vi "observacao.vi"() -> ()   [LabVIEW 2012] (continued)
                    n1498 = property on="Strong" class="Bool (strict)"("Disabled"=w1912) -> ()  [unwired: 2 in, 2 out]
                    n1499 = property on="WeakSel" class="Bool (strict)"("Value"=w1911) -> ()  [unwired: 2 in, 2 out]
                    n1500 = property on="MediumSel" class="Bool (strict)"("Value"=w1913) -> ()  [unwired: 2 in, 2 out]
                    n1501 = property on="StrongSel" class="Bool (strict)"("Value"=w1911) -> ()  [unwired: 2 in, 2 out]
                    n1502 = property on="Coude" class="Bool (strict)"("DisabledEnum"=w1912) -> ()  [unwired: 2 in, 2 out]
                    n1503 = property on="CoudeSel" class="Bool (strict)"("Value"=w1911) -> ()  [unwired: 2 in, 2 out]
                    n1504 = call "Monta Comando.vi"("Comando"=w1914, "Dispositivo"="FLAT_LO", "Controlador"=w1910) -> ()  [unwired: 4 in, 3 out]
                  }
                  frame True {
                    w1925 = FALSE ("Medium")
                    n1505 = Get Date/Time In Seconds() -> (seconds since 1Jan1904=w1928:timestamp)
                    n1506 = Add(x=w1928, y=10.0) -> (x+y=w1929:timestamp)
                    n1507 = local write "alarm Time"(w1929) -> ()
                    n1508 = property on="Mensage Alarme" class="Str"("Visible"=TRUE) -> ()  [unwired: 2 in, 2 out]
                    n1509 = local write "Flag Alarm"(TRUE ("Flag Alarm")) -> ()
                    n1510 = property on="Medium" class="Bool (strict)"("Value"=w1925) -> ()  [unwired: 2 in, 2 out]
                    n1511 = property on="MediumSel" class="Bool (strict)"("Value"=w1925) -> ()  [unwired: 2 in, 2 out]
                  }
                }
              }
              event "Strong": Value Change {
                w1932 = u16 6 items=["Alarme", "Atencao", "Erro", "Ocupado", "TBD", "LCB", "Trapeira", "Paravento", "DomoRap", "DomoCW", "DomoCCW", "TBD", "Em movimento", "TBD"] ("NomeStatus")
                n1512 = event-data() -> ("NewVal"=w1933:bool)  [unwired: 1 in, 5 out]
                n1513 = call "Bit Status CUP.vi"("NomeStatus"=w1932) -> ("StatBit"=w1931:bool)
                n1514 = case shown="False" w1931 {
                  tunnel: w1933 -> [w1941 _]
                  frame False {
                    w1934 = u16 4 items=["ZERO", "AH", "DEC", "TUBO", "CUP"] ("Controlador")
                    n1515 = case shown="True" w1941 {
                      tunnel: [FALSE w1949] -> w1936
                      tunnel: [w1942 w1949] -> w1940
                      tunnel: [0 2] -> w1937
                      tunnel: ["DESLIGAR" "LIGAR"] -> w1939
                      tunnel: [w1942 TRUE] -> w1938
                      frame False {
                        w1942 = FALSE
                      }
                      frame True {
                        w1949 = FALSE
                        n1516 = local write "DOME"(FALSE) -> ()
                        n1517 = local write "StatShutter"("Busy to Close" ("Status")) -> ()
                      }
                    }
                    n1518 = property on="Medium" class="Bool (strict)"("Disabled"=w1937) -> ()  [unwired: 2 in, 2 out]
                    n1519 = property on="Weak" class="Bool (strict)"("Disabled"=w1937) -> ()  [unwired: 2 in, 2 out]
                    n1520 = property on="Coude" class="Bool (strict)"("DisabledEnum"=w1937) -> ()  [unwired: 2 in, 2 out]
                    n1521 = property on="WeakSel" class="Bool (strict)"("Value"=w1940) -> ()  [unwired: 2 in, 2 out]
                    n1522 = property on="MediumSel" class="Bool (strict)"("Value"=w1936) -> ()  [unwired: 2 in, 2 out]
                    n1523 = property on="StrongSel" class="Bool (strict)"("Value"=w1938) -> ()  [unwired: 2 in, 2 out]
                    n1524 = property on="CoudeSel" class="Bool (strict)"("Value"=w1936) -> ()  [unwired: 2 in, 2 out]
                    n1525 = call "Monta Comando.vi"("Comando"=w1939, "Dispositivo"="FLAT_HI", "Controlador"=w1934) -> ()  [unwired: 4 in, 3 out]
                  }
                  frame True {
                    w1952 = FALSE ("Strong")
                    n1526 = Get Date/Time In Seconds() -> (seconds since 1Jan1904=w1955:timestamp)
                    n1527 = Add(x=w1955, y=10.0) -> (x+y=w1956:timestamp)
                    n1528 = local write "alarm Time"(w1956) -> ()
                    n1529 = property on="Mensage Alarme" class="Str"("Visible"=TRUE) -> ()  [unwired: 2 in, 2 out]
                    n1530 = local write "Flag Alarm"(TRUE ("Flag Alarm")) -> ()
                    n1531 = property on="StrongSel" class="Bool (strict)"("Value"=w1952) -> ()  [unwired: 2 in, 2 out]
                    n1532 = property on="Strong" class="Bool (strict)"("Value"=w1952) -> ()  [unwired: 2 in, 2 out]
                  }
                }
              }
              event "Coude": Value Change {
                w1959 = u16 6 items=["Alarme", "Atencao", "Erro", "Ocupado", "TBD", "LCB", "Trapeira", "Paravento", "DomoRap", "DomoCW", "DomoCCW", "TBD", "Em movimento", "TBD"] ("NomeStatus")
                n1533 = event-data() -> ("NewVal"=w1960:bool)  [unwired: 1 in, 5 out]
                n1534 = call "Bit Status CUP.vi"("NomeStatus"=w1959) -> ("StatBit"=w1958:bool)
                n1535 = case shown="False" w1958 {
                  tunnel: w1960 -> [w1967 _]
                  frame False {
                    w1961 = u16 4 items=["ZERO", "AH", "DEC", "TUBO", "CUP"] ("Controlador")
                    n1536 = case shown="True" w1967 {
                      tunnel: [FALSE w1976] -> w1964
                      tunnel: [w1969 w1976] -> w1965
                      tunnel: [0 2] -> w1963
                      tunnel: ["DESLIGAR" "LIGAR"] -> w1968
                      tunnel: [w1969 TRUE] -> w1966
                      frame False {
                        w1969 = FALSE
                      }
                      frame True {
                        w1976 = FALSE
                        n1537 = local write "DOME"(FALSE) -> ()
                        n1538 = local write "StatShutter"("Busy to Close" ("Status")) -> ()
                      }
                    }
                    n1539 = property on="StrongSel" class="Bool (strict)"("Value"=w1965) -> ()  [unwired: 2 in, 2 out]
                    n1540 = property on="CoudeSel" class="Bool (strict)"("Value"=w1966) -> ()  [unwired: 2 in, 2 out]
                    n1541 = property on="MediumSel" class="Bool (strict)"("Value"=w1964) -> ()  [unwired: 2 in, 2 out]
                    n1542 = property on="Weak" class="Bool (strict)"("DisabledEnum"=w1963) -> ()  [unwired: 2 in, 2 out]
                    n1543 = property on="Medium" class="Bool (strict)"("DisabledEnum"=w1963) -> ()  [unwired: 2 in, 2 out]
                    n1544 = property on="Strong" class="Bool (strict)"("DisabledEnum"=w1963) -> ()  [unwired: 2 in, 2 out]
                    n1545 = property on="WeakSel" class="Bool (strict)"("Value"=w1964) -> ()  [unwired: 2 in, 2 out]
                    n1546 = call "Monta Comando.vi"("Comando"=w1968, "Dispositivo"="FLAT_COUDE", "Controlador"=w1961) -> ()  [unwired: 4 in, 3 out]
                  }
                  frame True {
                    w1979 = FALSE ("Coude")
                    n1547 = Get Date/Time In Seconds() -> (seconds since 1Jan1904=w1982:timestamp)
                    n1548 = Add(x=w1982, y=10.0) -> (x+y=w1983:timestamp)
                    n1549 = local write "alarm Time"(w1983) -> ()
                    n1550 = property on="Mensage Alarme" class="Str"("Visible"=TRUE) -> ()  [unwired: 2 in, 2 out]
                    n1551 = local write "Flag Alarm"(TRUE ("Flag Alarm")) -> ()
                    n1552 = property on="CoudeSel" class="Bool (strict)"("Value"=w1979) -> ()  [unwired: 2 in, 2 out]
                    n1553 = property on="Coude" class="Bool (strict)"("Value"=w1979) -> ()  [unwired: 2 in, 2 out]
                  }
                }
              }
            }
            n1554 = disable-structure shown="Disabled" {
              frame Disabled {
                w1879 = u16 4 items=["ZERO", "AH", "DEC", "TUBO", "CUP"] ("Controlador")
                n1555 = call "Monta Comando.vi"("Comando"="FECHAR", "Dispositivo"="TRAPEIRA" ("Comando"), "Controlador"=w1879) -> ()  [unwired: 4 in, 3 out]
              }
              frame Enabled {
              }
            }
          }
          frame "LIST" {
            n1556 = stacked-sequence {
              frame #0 {
                # "Muda nome do controle de RA para AH se MAFmax == 100"
                n1557 = case shown="True" "SET coord" {
                  frame False {
                  }
                  frame True {
                    n1558 = stacked-sequence {
                      frame #0 {
                        w2000 = "2000"
                        # "Valores aux para Detectar Edição"
                        n1559 = local read "Multicolumn Listbox"() -> (w2007:i32[])
                        n1560 = property on="Multicolumn Listbox" class="MCListbox (strict)"() -> ("Item Names"=w2005:string[][])  [unwired: 2 in, 2 out]
                        n1561 = Index Array(array=w2007, index=0) -> (element=w2004:i32)
                        n1562 = local write "FLAG SET COORD"(TRUE ("FLAG_MAG")) -> ()
                        n1563 = Index Array(array=w2005, index (row)=w2004) -> (element=w2003:string[])  [unwired: 1 in]
                        n1564 = Index Array(array=w2003, index #1=0 ("index")) -> (element #1=w1996:string, element #2=w1994:string, element #3=w1995:string, element #4=w1997:string, element #5=w1999:string, element #6=w1998:string)  [unwired: 5 in]
                        "RA AUX" <- w1994
                        "AUX EDITA Name" <- w1996
                        "AUX EDITA RA" <- w1994
                        "AUX EDITA DEC" <- w1995
                        "AUX EDITA PMRA" <- w1999
                        "AUX EDITA PMDEC" <- w1998
                        n1565 = local write "StrPointObjPMRA"(w1999) -> ()
                        n1566 = local write "StrPointObjPMDEC"(w1998) -> ()
                        n1567 = local write "StrPointObjName"(w1996) -> ()
                        n1568 = local write "StrPointObjRA"(w1994) -> ()
                        n1569 = local write "StrPointObjDEC"(w1995) -> ()
                        n1570 = local write "MAG"(w1997) -> ()
                        n1571 = local write "StrPointObjEpoch"(w2000) -> ()
                        "EPOCH AUX" <- w2000
                        "AUX EDITA EPOCH" <- w2000
                      }
                      frame #1 {
                        n1572 = case shown="True" "Case Constant\n(See Context Help) 7" {
                          frame False {
                          }
                          frame True {
                            # "Ao clicar SET COORD, fechar a aba LIST e abrir a aba POINTING"
                            n1573 = local write "Setup, Pointing & Guiding"(T2."POINTING" ("Setup, Pointing & Guiding")) -> ()
                          }
                        }
                      }
                    }
                  }
                }
                n1574 = case shown="True" "Clear ALL" {
                  frame False {
                  }
                  frame True {
                    n1575 = Two Button Dialog(message="Will you clear All Table?") -> (T button?=w2010:bool)  [unwired: 2 in]
                    n1576 = case shown="True" w2010 {
                      frame False {
                      }
                      frame True {
                        w2012 = string[][] [] ("Item Names")
                        # "Limpa a Tabela Inteira"
                        n1577 = property on="Multicolumn Listbox" class="MCListbox (strict)"("Item Names"=w2012) -> ()  [unwired: 2 in, 2 out]
                        n1578 = local write "subarray"(w2012) -> ()
                      }
                    }
                  }
                }
                n1579 = local read "MAG Max"() -> (w1986:dbl)
                n1580 = Equal?(x=100.0, y=w1986) -> (x = y?=w1985:bool)
                n1581 = case shown="False" w1985 {
                  frame False {
                    n1582 = flat-sequence {
                      frame #0 {
                        w1990 = FALSE
                        n1583 = property on="RA Max" class="DigNum (strict)"("Caption.Visible"=w1990) -> ()  [unwired: 2 in, 2 out]
                        n1584 = property on="RA Min" class="DigNum (strict)"("Caption.Visible"=w1990) -> ()  [unwired: 2 in, 2 out]
                      }
                      frame #1 {
                        w1991 = TRUE
                        n1585 = property on="RA Min" class="DigNum (strict)"("Label.Visible"=w1991) -> ()  [unwired: 2 in, 2 out]
                        n1586 = property on="RA Max" class="DigNum (strict)"("Label.Visible"=w1991) -> ()  [unwired: 2 in, 2 out]
                      }
                    }
                  }
                  frame True {
                    n1587 = flat-sequence {
                      frame #0 {
                        w1992 = FALSE
                        n1588 = property on="RA Max" class="DigNum (strict)"("Label.Visible"=w1992) -> ()  [unwired: 2 in, 2 out]
                        n1589 = property on="RA Min" class="DigNum (strict)"("Label.Visible"=w1992) -> ()  [unwired: 2 in, 2 out]
                      }
                      frame #1 {
                        w1993 = TRUE
                        n1590 = property on="RA Min" class="DigNum (strict)"("Caption.Visible"=w1993) -> ()  [unwired: 2 in, 2 out]
                        n1591 = property on="RA Max" class="DigNum (strict)"("Caption.Visible"=w1993) -> ()  [unwired: 2 in, 2 out]
                      }
                    }
                  }
                }
              }
              frame #1 {
                # "MUDANÇA:\nUPLOAD carrega\ncatálogo usuário"
                n1592 = case shown="True" "Upload" {
                  frame False {
                  }
                  frame True {
                    n1593 = File Dialog() -> (0:w2018:errorcluster, 1:w2020:bool, 3:w2019:path)  [unwired: 7 in, 1 out]
                    n1594 = Unbundle(w2018) -> ("status"=w2017:bool)  [unwired: 2 out]
                    n1595 = Not(x=w2017) -> (.not. x?=w2015:bool)
                    n1596 = And(x=w2020, y=w2015) -> (x .and. y?=w2016:bool)
                    n1597 = case shown="False" w2016 {
                      tunnel: w2019 -> [w2023 _]
                      frame False {
                        w2024 = 0 ("Slide")
                        # "Abre Arquivo Escolhido"
                        n1598 = Strip Path(path=w2023) -> (name=w2021:string)  [unwired: 1 out]
                        n1599 = Path To String(path=w2023) -> (string=w2028:string)
                        n1600 = local write "List File"(w2021) -> ()
                        n1601 = call "leexel.vi"("path"=w2028) -> ("array 5"=w2022:string[][])  [unwired: 4 in]
                        n1602 = local write "Slide"(w2024) -> ()
                        n1603 = local write "subarray"(w2022) -> ()
                        n1604 = Array Subset(array=w2022, index (row)=w2024, length (row)=10 ("length"), index (col)=w2024, length (col)=8 ("index")) -> (w2025:string[][])
                        n1605 = property on="Multicolumn Listbox" class="MCListbox (strict)"("Item Names"=w2025) -> ()  [unwired: 2 in, 2 out]
                      }
                      frame True {
                      }
                    }
                  }
                }
                n1606 = case shown="True" "Save AS" {
                  frame False {
                  }
                  frame True {
                    n1607 = File Dialog() -> (0:w2029:errorcluster, 1:w2031:bool, 3:w2030:path)  [unwired: 7 in, 1 out]
                    n1608 = Unbundle(w2029) -> ()  [unwired: 3 out]
                    n1609 = case shown="False" w2031 {
                      tunnel: w2030 -> [w2033 _]
                      frame False {
                        # "Salva Arquivo Escolhido"
                        n1610 = Path To String(path=w2033) -> (string=w2034:string)
                        n1611 = case shown="True" "Case Constant\n(See Context Help) 8" {
                          tunnel: w2034 -> [_ w2036]
                          frame False {
                          }
                          frame True {
                            n1612 = local read "subarray"() -> (w2035:string[][])
                            n1613 = call "salvaexel.vi"("appended array"=w2035, "file name p/ exell"=w2036) -> ()  [unwired: 1 in, 1 out]
                          }
                        }
                      }
                      frame True {
                      }
                    }
                  }
                }
              }
              frame #2 {
                # "Acerta Posição do Slide"
                n1614 = local read "Tot Linhas"() -> (w2041:i32)
                n1615 = Multiply(x="Slide", y=w2041) -> (x*y=w2040:dbl)
                n1616 = Divide(x=w2040, y=24.0) -> (x/y=w2038:dbl)
                n1617 = case shown="True" "Save" {
                  frame False {
                  }
                  frame True {
                    w2092 = "C:\\TCS\\ARQUIVOS\\List.lst"
                    # "Cria e Lê arquivo\nonde voce está\ntrabalhando"
                    n1618 = String To Path(string=w2092) -> (path=w2091:path)
                    n1619 = stacked-sequence {
                      tunnel: w2091 -> [w2093 _]
                      tunnel: w2092 -> [_ w2095]
                      frame #0 {
                        # "Apaga o arquivo"
                        n1620 = Delete(path (use dialog)=w2093) -> ()  [unwired: 4 in, 3 out]
                      }
                      frame #1 {
                        # "Salva a lista"
                        n1621 = local read "subarray"() -> (w2094:string[][])
                        n1622 = call "salvaexel.vi"("appended array"=w2094, "file name p/ exell"=w2095) -> ()  [unwired: 1 in, 1 out]
                      }
                    }
                  }
                }
                n1623 = Not Equal?(x=w2038, y="Slide old") -> (x != y?=w2044:bool)
                n1624 = case shown="True" "Open BSC" {
                  frame False {
                  }
                  frame True {
                    n1625 = stacked-sequence {
                      frame #0 {
                        w2097 = FALSE
                        # "MUDANÇA:\nUPLOAD carrega\ncatálogo usuário"
                        # "Faz Aparecer os Botões"
                        n1626 = property on="Delete" class="Bool"("Visible"=w2097) -> ()  [unwired: 2 in, 2 out]
                        n1627 = property on="EDIT" class="Bool"("Visible"=w2097) -> ()  [unwired: 2 in, 2 out]
                        n1628 = property on="Clear ALL" class="Bool"("Visible"=w2097) -> ()  [unwired: 2 in, 2 out]
                        n1629 = property on="Save AS" class="Bool"("Visible"=w2097) -> ()  [unwired: 2 in, 2 out]
                        n1630 = property on="Save" class="Bool"("Visible"=w2097) -> ()  [unwired: 2 in, 2 out]
                        n1631 = property on="Insert" class="Bool"("Visible"=w2097) -> ()  [unwired: 2 in, 2 out]
                        n1632 = property on="Upload" class="Bool"("Visible"=TRUE) -> ()  [unwired: 2 in, 2 out]
                      }
                      frame #1 {
                        w2105 = 0 ("Slide")
                        w2099 = "C:\\TCS\\ARQUIVOS\\BSC_08.txt"
                        # "Cria e Lê arquivo\nonde voce está\ntrabalhando"
                        n1633 = local write "Slide"(w2105) -> ()
                        n1634 = call "leexel.vi"("path"=w2099) -> ("array 5"=w2103:string[][])  [unwired: 4 in]
                        "subarray" <- w2103
                        n1635 = Array Subset(array=w2103, index (row)=w2105, length (row)=11 ("length"), index (col)=w2105, length (col)=8 ("index")) -> (w2106:string[][])
                        n1636 = Array Size(array=w2103) -> (size(s)=w2104:i32[])
                        n1637 = String To Path(string=w2099) -> (path=w2100:path)
                        n1638 = property on="Multicolumn Listbox" class="MCListbox (strict)"("Item Names"=w2106) -> ()  [unwired: 2 in, 2 out]
                        n1639 = Strip Path(path=w2100) -> (name=→"List File":string)  [unwired: 1 out]
                        n1640 = Index Array(array=w2104, index=0) -> (element=→"Tot Linhas":i32)
                        "Saida Path string" <- w2099
                      }
                      frame #2 {
                        n1641 = local read "Tot Linhas"() -> (w2117:i32)
                        n1642 = Quotient & Remainder(x=10000, y=w2117) -> (floor(x/y)=w2115:i32)  [unwired: 1 out]
                        n1643 = Divide(x=w2115, y=1000) -> (x/y=w2112:dbl)
                        n1644 = Multiply(x=w2112, y=24.0) -> (x*y=w2113:dbl)
                        n1645 = property on="Slide" class="Slide (strict)"("Data Entry Limits:Increment"=w2113) -> ()  [unwired: 2 in, 2 out]
                        "ScaleMax" <- "24" ("ScaleMax")
                        "ScaleMin" <- "0" ("ScaleMin")
                      }
                    }
                  }
                }
                n1646 = case shown="True" w2044 {
                  tunnel: w2038 -> [_ w2049]
                  frame False {
                  }
                  frame True {
                    n1647 = stacked-sequence {
                      seq-local: [w2053 _] -> [_ w2058]
                      tunnel: w2049 -> [w2054 _]
                      frame #0 {
                        # "Previne estouro\nda planilha"
                        n1648 = local read "Tot Linhas"() -> (w2052:i32)
                        n1649 = Subtract(x=w2052, y=10) -> (x-y=w2050:i32)
                        n1650 = Greater Or Equal?(x=w2054, y=w2050) -> (x >= y?=w2055:bool)
                        n1651 = case shown="False" w2055 {
                          tunnel: [w2056 w2057] -> w2053
                          tunnel: w2050 -> [_ w2057]
                          tunnel: w2054 -> [w2056 _]
                          frame False {
                          }
                          frame True {
                          }
                        }
                      }
                      frame #1 {
                        n1652 = local read "subarray"() -> (w2060:string[][])
                        n1653 = local write "Slide old"(w2058) -> ()
                        n1654 = Array Subset(array=w2060, index (row)=w2058, length (row)=11 ("length"), index (col)=0 ("index"), length (col)=8 ("index")) -> (w2059:string[][])
                        n1655 = property on="Multicolumn Listbox" class="MCListbox (strict)"("Item Names"=w2059) -> ()  [unwired: 2 in, 2 out]
                      }
                    }
                  }
                }
                n1656 = property on="Multicolumn Listbox" class="MCListbox (strict)"("Selection Color"=u32 10336195) -> ()  [unwired: 2 in, 2 out]
                n1657 = case shown="True" "Delete" {
                  frame False {
                  }
                  frame True {
                    n1658 = local read "Multicolumn Listbox"() -> (w2070:i32[])
                    n1659 = Index Array(array=w2070, index=0) -> (element=w2064:i32)
                    n1660 = Number To Decimal String(number=w2064) -> (decimal integer string=w2067:string)  [unwired: 1 in]
                    n1661 = Concatenate Strings("Delete Line Number: " ("string"), w2067) -> (w2065:string)
                    n1662 = Two Button Dialog(message=w2065) -> (T button?=w2066:bool)  [unwired: 2 in]
                    n1663 = case shown="True" w2066 {
                      tunnel: w2064 -> [_ w2071]
                      frame False {
                      }
                      frame True {
                        n1664 = stacked-sequence {
                          tunnel: w2071 -> [w2075 _]
                          frame #0 {
                            # "Apaga a Coluna Escolhida"
                            n1665 = property on="Multicolumn Listbox" class="MCListbox (strict)"() -> ("Item Names"=w2078:string[][])  [unwired: 2 in, 2 out]
                            n1666 = local read "Slide"() -> (w2076:dbl)
                            n1667 = local read "subarray"() -> (w2073:string[][])
                            n1668 = Add(x=w2075, y=w2076) -> (x+y=w2074:dbl)
                            n1669 = Delete From Array(array=w2078, index (row)=w2075) -> (array with subset deleted=w2077:string[][])  [unwired: 2 in, 1 out]
                            n1670 = Delete From Array(array=w2073, index (row)=w2074) -> (array with subset deleted=w2072:string[][])  [unwired: 2 in, 1 out]
                            n1671 = local write "subarray"(w2072) -> ()
                            n1672 = property on="Multicolumn Listbox" class="MCListbox (strict)"("Item Names"=w2077) -> ()  [unwired: 2 in, 2 out]
                          }
                          frame #1 {
                            # "Volta para a coluna Zero"
                            n1673 = local write "Multicolumn Listbox"(i32[] [0] ("Multicolumn Listbox")) -> ()
                          }
                        }
                      }
                    }
                  }
                }
                n1674 = case shown="True" "Insert" {
                  frame False {
                  }
                  frame True {
                    n1675 = stacked-sequence {
                      seq-local: [w2081 _ _] -> [_ w2083 _]
                      seq-local: [w2080 _ _] -> [_ w2082 _]
                      frame #0 {
                        n1676 = call "Tela_Set_Coordenadas.vi"() -> ("Saída"=w2081:bool, "Val Saída"=w2080:string[])  [unwired: 4 in]
                      }
                      frame #1 {
                        n1677 = case shown="True" w2083 {
                          tunnel: w2082 -> [_ w2084]
                          frame False {
                          }
                          frame True {
                            # "Insere Linha Preenchida"
                            n1678 = local read "subarray"() -> (w2086:string[][])
                            n1679 = property on="Multicolumn Listbox" class="MCListbox (strict)"() -> ("Item Names"=w2088:string[][])  [unwired: 2 in, 2 out]
                            n1680 = Build Array (concatenate)(w2088, w2084) -> (w2087:string[][])
                            n1681 = Build Array (concatenate)(w2086, w2084) -> (w2085:string[][])
                            n1682 = property on="Multicolumn Listbox" class="MCListbox (strict)"("Item Names"=w2087) -> ()  [unwired: 2 in, 2 out]
                            n1683 = local write "subarray"(w2085) -> ()
                          }
                        }
                      }
                      frame #2 {
                        # "Depois de inserir um novo objeto na tabela,\n com o comando INSERT, mudar o objeto \nselecionado para esse novo registro."
                        n1684 = property on="Multicolumn Listbox" class="MCListbox (strict)"() -> ("Number of Rows"=w2090:u32)  [unwired: 2 in, 2 out]
                        n1685 = Build Array(w2090) -> (w2089:u32[])
                        n1686 = local write "Multicolumn Listbox"(w2089) -> ()
                      }
                    }
                  }
                }
              }
              frame #3 {
                # "Editar a Lista"
                n1687 = case shown="True" "Open" {
                  frame False {
                  }
                  frame True {
                    n1688 = stacked-sequence {
                      frame #0 {
                        w2120 = TRUE
                        # "Faz Aparecer os Botões"
                        n1689 = property on="Delete" class="Bool"("Visible"=w2120) -> ()  [unwired: 2 in, 2 out]
                        n1690 = property on="EDIT" class="Bool"("Visible"=w2120) -> ()  [unwired: 2 in, 2 out]
                        n1691 = property on="Clear ALL" class="Bool"("Visible"=w2120) -> ()  [unwired: 2 in, 2 out]
                        n1692 = property on="Upload" class="Bool"("Visible"=w2120) -> ()  [unwired: 2 in, 2 out]
                        n1693 = property on="Save AS" class="Bool"("Visible"=w2120) -> ()  [unwired: 2 in, 2 out]
                        n1694 = property on="Save" class="Bool"("Visible"=w2120) -> ()  [unwired: 2 in, 2 out]
                        n1695 = property on="Insert" class="Bool"("Visible"=w2120) -> ()  [unwired: 2 in, 2 out]
                      }
                      frame #1 {
                        w2128 = 0 ("Slide")
                        w2124 = "C:\\TCS\\ARQUIVOS\\List.lst"
                        n1696 = local write "Saida Path string"(w2124) -> ()
                        n1697 = local write "Slide"(w2128) -> ()
                        n1698 = String To Path(string=w2124) -> (path=w2131:path)
                        n1699 = call "leexel.vi"("path"=w2124) -> ("array 5"=w2123:string[][])  [unwired: 4 in]
                        n1700 = Strip Path(path=w2131) -> (name=w2130:string)  [unwired: 1 out]
                        n1701 = local write "subarray"(w2123) -> ()
                        n1702 = local write "List File"(w2130) -> ()
                        n1703 = Array Subset(array=w2123, index (row)=w2128, length (row)=10 ("length"), index (col)=w2128, length (col)=8 ("index")) -> (w2127:string[][])
                        n1704 = Array Size(array=w2123) -> (size(s)=w2121:i32[])
                        n1705 = property on="Multicolumn Listbox" class="MCListbox (strict)"("Item Names"=w2127) -> ()  [unwired: 2 in, 2 out]
                        n1706 = Index Array(array=w2121, index=0) -> (element=w2122:i32)
                        n1707 = local write "Tot Linhas"(w2122) -> ()
                      }
                      frame #2 {
                        w2132 = ""
                        n1708 = local read "Tot Linhas"() -> (w2139:i32)
                        n1709 = Quotient & Remainder(x=10000, y=w2139) -> (floor(x/y)=w2137:i32)  [unwired: 1 out]
                        n1710 = Divide(x=w2137, y=1000) -> (x/y=w2134:dbl)
                        n1711 = Multiply(x=w2134, y=24.0) -> (x*y=w2135:dbl)
                        n1712 = local write "ScaleMin"(w2132) -> ()
                        n1713 = local write "ScaleMax"(w2132) -> ()
                        n1714 = property on="Slide" class="Slide (strict)"("Data Entry Limits:Increment"=w2135) -> ()  [unwired: 2 in, 2 out]
                      }
                    }
                  }
                }
                n1715 = case shown="True" "EDIT" {
                  frame False {
                  }
                  frame True {
                    (unwired) "Edit the marked Line and soon after presses SAVE"
                    n1716 = call "Edita_lista.vi"() -> ("lista Auxiliar"=w2140:string[][])  [unwired: 5 in]
                    n1717 = property on="Multicolumn Listbox" class="MCListbox (strict)"("Item Names"=w2140) -> ()  [unwired: 2 in, 2 out]
                  }
                }
              }
              frame #4 {
                n1718 = case shown="True" "Filter RA" {
                  frame False {
                  }
                  frame True {
                    n1719 = while {
                      shift-right: [w2143] -> _
                      shift-left: "inicio" -> [w2145]
                      stop <- w2144 stop-if-true
                      n1720 = case shown="\"filtra\"" w2145 {
                        tunnel: [FALSE w2195 TRUE TRUE] -> w2144
                        tunnel: [w2165 w2196 "fim" "fim"] -> w2143
                        frame "inicio" {
                          # "RAmin"
                          # "RAmax"
                          # "Testa se:\n| Ramax - Ramin | >=1\n|Decmax -Decmin | >=1\n|Magmax -Magmin | >=1"
                          n1721 = local read "MAG Max"() -> (w2159:dbl)
                          n1722 = local read "MAG Min"() -> (w2174:dbl)
                          n1723 = Equal?(x=100.0, y=w2159) -> (x = y?=w2151:bool)
                          n1724 = Subtract(x=w2159, y=w2174) -> (x-y=w2171:dbl)
                          n1725 = case shown="True" w2151 {
                            tunnel: "RA Min" -> [w2179 w2187]
                            tunnel: [w2179 w2186] -> w2146
                            tunnel: "RA Max" -> [w2178 w2188]
                            tunnel: [w2178 w2183] -> w2147
                            frame False {
                            }
                            frame True {
                              w2192 = 24 ("RA Max")
                              # "12h/PI()"
                              # "TS, rad"
                              # "TS, hora"
                              # "RAmin"
                              # "RAmax"
                              # "AHmax"
                              # "AHmin"
                              # "MUDANÇA 7/4/2011:\nSe MAGmax >= 100,\ntratar RA como AH."
                              n1726 = global read "Global_Telescopio.vi" "Sideral Time"() -> (w2182:dbl)
                              n1727 = Multiply(x=w2182, y=3.8197) -> (x*y=w2181:dbl)
                              n1728 = To Long Integer(number=w2181) -> (32bit integer=w2189:i32)
                              n1729 = Subtract(x=w2189, y=w2188) -> (x-y=w2185:i32)
                              n1730 = Subtract(x=w2189, y=w2187) -> (x-y=w2184:i32)
                              n1731 = Add(x=w2192, y=w2185) -> (x+y=w2191:i32)
                              n1732 = Less Than 0?(x=w2185) -> (x < 0?=w2194:bool)
                              n1733 = Add(x=w2192, y=w2184) -> (x+y=w2190:i32)
                              n1734 = Less Than 0?(x=w2184) -> (x < 0?=w2193:bool)
                              n1735 = Select(t=w2191, s=w2194, f=w2185) -> (s? t:f=w2186:i32)
                              n1736 = Select(t=w2190, s=w2193, f=w2184) -> (s? t:f=w2183:i32)
                            }
                          }
                          n1737 = Less?(x=w2171, y=1.0) -> (x < y?=w2168:bool)
                          n1738 = local read "DEC Max"() -> (w2176:i32)
                          n1739 = local read "DEC Min"() -> (w2175:i32)
                          n1740 = local write "RA Min 2"(w2146) -> ()
                          n1741 = local write "RA Max 2"(w2147) -> ()
                          n1742 = Less?(x=w2147, y=w2146) -> (x < y?=w2152:bool)
                          "FiltroDuplo" <- w2152
                          n1743 = Equal?(x=w2147, y=w2146) -> (x = y?=w2150:bool)
                          n1744 = Add(x=w2147, y=24 ("RA Max")) -> (x+y=w2156:i32)
                          n1745 = Subtract(x=w2156, y=w2146) -> (x-y=w2155:i32)
                          n1746 = Subtract(x=w2176, y=w2175) -> (x-y=w2173:i32)
                          n1747 = Greater?(x=w2155, y=12) -> (0:w2153:bool)
                          n1748 = Less?(x=w2173, y=1) -> (x < y?=w2169:bool)
                          n1749 = And(x=w2153, y=w2152) -> (x .and. y?=w2160:bool)
                          n1750 = control-ref of="Erro"() -> (w2162:refnum<vi>)
                          n1751 = Compound Arithmetic op=OR(w2160, w2150, w2169, w2168) -> (w2167:bool)
                          n1752 = property class="Bool (strict)"(reference=w2162, "Boolean Text.Text"="WAIT") -> ()  [unwired: 1 in, 2 out]
                          n1753 = Select(t="erro", s=w2167, f="filtra") -> (s? t:f=w2165:string)
                          "Erro" <- FALSE ("Fim")
                        }
                        frame "filtra" {
                          n1754 = stacked-sequence {
                            seq-local: [w2200 _ _ _] -> [_ w2243 _ _]
                            seq-local: [_ w2244 _ _] -> [_ _ w2263 _]
                            seq-local: [_ _ w2264 _] -> [_ _ _ w2289]
                            tunnel: [_ _ _ "fim"] -> w2196
                            tunnel: [_ _ _ FALSE] -> w2195
                            frame #0 {
                              n1755 = property on="EDIT" class="Bool"() -> ("Visible"=w2197:bool)  [unwired: 2 in, 2 out]
                              n1756 = case shown="True" w2197 {
                                tunnel: ["C:\\TCS\\ARQUIVOS\\BSC_08.txt" "C:\\TCS\\ARQUIVOS\\List.lst"] -> w2199
                                frame False {
                                }
                                frame True {
                                }
                              }
                              n1757 = call "leexel.vi"("path"=w2199) -> ("array 5"=w2198:string[][])  [unwired: 4 in]
                              n1758 = Index Array(array=w2198, index (col)=1 ("disabled index (col)")) -> (element=w2202:string[])  [unwired: 1 in]
                              n1759 = for {
                                tunnel: w2202 -> [w2218] mode=indexing
                                shift-right: [w2212] -> w2200
                                shift-left: string[][] [] ("Item Names") -> [w2214]
                                tunnel: w2198 -> [w2211] mode=indexing
                                # "Filtro de RA"
                                n1760 = local read "FiltroDuplo"() -> (w2210:bool)
                                n1761 = String Subset(string=w2218, offset (0)=0, length (rest)=2 ("length (rest)")) -> (substring=w2215:string)
                                n1762 = Decimal String To Number(string=w2215) -> (number=w2209:i32)  [unwired: 2 in, 1 out]
                                n1763 = case shown="False" w2210 {
                                tunnel: "RA Max 2" -> [w2223 w2228]
                                tunnel: "RA Min 2" -> [w2222 w2225]
                                tunnel: [w2221 w2230] -> w2213
                                tunnel: w2209 -> [w2220 w2229]
                                tunnel: [FALSE w2224] -> w2208
                                frame False {
                                n1764 = In Range and Coerce(upper limit=w2223, x=w2220, lower limit=w2222) -> (In Range?=w2221:bool)  [unwired: 1 out]
                                }
                                frame True {
                                n1765 = In Range and Coerce(upper limit=w2228, x=w2229, lower limit=0 ("upper limit")) -> (In Range?=w2231:bool)  [unwired: 1 out]
                                n1766 = In Range and Coerce(upper limit=24 ("lower limit"), x=w2229, lower limit=w2225) -> (In Range?=w2224:bool)  [unwired: 1 out]
                                n1767 = Or(x=w2231, y=w2224) -> (x .or. y?=w2230:bool)
                                }
                                }
                                n1768 = case shown="True" w2213 {
                                tunnel: w2214 -> [w2232 w2236]
                                tunnel: [w2232 w2235] -> w2212
                                tunnel: w2211 -> [_ w2234]
                                tunnel: w2208 -> [_ w2233]
                                frame False {
                                }
                                frame True {
                                n1769 = case shown="False" w2233 {
                                tunnel: w2236 -> [w2239 w2241]
                                tunnel: [w2238 w2240] -> w2235
                                tunnel: w2234 -> [w2237 w2242]
                                frame False {
                                n1770 = Build Array (concatenate)(w2239, w2237) -> (w2238:string[][])
                                }
                                frame True {
                                n1771 = Build Array (concatenate)(w2242, w2241) -> (w2240:string[][])
                                }
                                }
                                }
                                }
                              }
                            }
                            frame #1 {
                              # "Filtro de DEC"
                              n1772 = Index Array(array=w2243, index (col)=2 ("disabled index (col)")) -> (element=w2246:string[])  [unwired: 1 in]
                              n1773 = for {
                                tunnel: w2246 -> [w2258] mode=indexing
                                shift-right: [w2251] -> w2244
                                shift-left: string[][] [] ("Item Names") -> [w2253]
                                tunnel: w2243 -> [w2250] mode=indexing
                                n1774 = String Subset(string=w2258, offset (0)=0, length (rest)=3 ("length (rest)")) -> (substring=w2255:string)
                                n1775 = Decimal String To Number(string=w2255) -> (number=w2254:i32)  [unwired: 2 in, 1 out]
                                n1776 = In Range and Coerce(upper limit="DEC Max", x=w2254, lower limit="DEC Min") -> (In Range?=w2252:bool)  [unwired: 1 out]
                                n1777 = case shown="True" w2252 {
                                tunnel: w2253 -> [w2259 w2262]
                                tunnel: [w2259 w2261] -> w2251
                                tunnel: w2250 -> [_ w2260]
                                frame False {
                                }
                                frame True {
                                n1778 = Build Array (concatenate)(w2262, w2260) -> (w2261:string[][])
                                }
                                }
                              }
                            }
                            frame #2 {
                              # "Filtro de MAG"
                              n1779 = Index Array(array=w2263, index (col)=3 ("disabled index (col)")) -> (element=w2266:string[])  [unwired: 1 in]
                              n1780 = for {
                                tunnel: w2266 -> [w2268] mode=indexing
                                shift-right: [w2272] -> w2264
                                shift-left: string[][] [] ("Item Names") -> [w2276]
                                tunnel: w2263 -> [w2274] mode=indexing
                                n1781 = Fract/Exp String To Number(use system decimal point (T)=FALSE, string=w2268) -> (number=w2271:dbl)  [unwired: 2 in, 1 out]
                                n1782 = In Range and Coerce(upper limit="MAG Max", x=w2271, lower limit="MAG Min") -> (In Range?=w2275:bool)  [unwired: 1 out]
                                n1783 = case shown="True" w2275 {
                                tunnel: w2276 -> [w2277 w2280]
                                tunnel: [w2277 w2279] -> w2272
                                tunnel: w2274 -> [_ w2278]
                                frame False {
                                }
                                frame True {
                                n1784 = Build Array (concatenate)(w2280, w2278) -> (w2279:string[][])
                                }
                                }
                              }
                            }
                            frame #3 {
                              w2281 = 0 ("index")
                              n1785 = local write "subarray"(w2289) -> ()
                              n1786 = Array Size(array=w2289) -> (size(s)=w2301:i32[])
                              n1787 = Index Array(array=w2301, index=0) -> (element=w2294:i32)
                              n1788 = local write "Tot Linhas"(w2294) -> ()
                              n1789 = local write "Slide old"(w2281) -> ()
                              n1790 = local write "Slide"(w2281) -> ()
                              n1791 = Array Subset(array=w2289, index (row)=w2281, length (row)=11 ("length"), index (col)=0 ("index"), length (col)=8 ("index")) -> (w2290:string[][])
                              n1792 = property on="Multicolumn Listbox" class="MCListbox (strict)"("Item Names"=w2290) -> ()  [unwired: 2 in, 2 out]
                              n1793 = Quotient & Remainder(x=10000, y=w2294) -> (floor(x/y)=w2298:i32)  [unwired: 1 out]
                              n1794 = Divide(x=w2298, y=1000) -> (x/y=w2296:dbl)
                              n1795 = Multiply(x=w2296, y=24.0) -> (x*y=w2283:dbl)
                              n1796 = Decrement(x=w2283) -> (x-1=w2282:dbl)
                              n1797 = control-ref of="Erro"() -> (w2285:refnum<vi>)
                              n1798 = property class="Bool (strict)"(reference=w2285, "Boolean Text.Text"="") -> ()  [unwired: 1 in, 2 out]
                              n1799 = property on="Slide" class="Slide (strict)"("Data Entry Limits:Increment"=w2282) -> ()  [unwired: 2 in, 2 out]
                              n1800 = local write "Erro"(FALSE ("Erro")) -> ()
                            }
                          }
                        }
                        frame "erro", Default {
                          n1801 = control-ref of="Erro"() -> (w2303:refnum<vi>)
                          n1802 = property class="Bool (strict)"(reference=w2303, "Boolean Text.Text"="ERROR") -> ()  [unwired: 1 in, 2 out]
                          n1803 = local write "Erro"(TRUE ("Erro")) -> ()
                        }
                        frame "fim" {
                          n1804 = local read "RA Max 2"() -> (w2308:i32)
                          n1805 = local read "RA Min 2"() -> (w2307:i32)
                          n1806 = Number To Decimal String(number=w2307) -> (decimal integer string=w2310:string)  [unwired: 1 in]
                          n1807 = Number To Decimal String(number=w2308) -> (decimal integer string=w2309:string)  [unwired: 1 in]
                          n1808 = local write "ScaleMin"(w2310) -> ()
                          n1809 = local write "ScaleMax"(w2309) -> ()
                        }
                      }
                    }
                  }
                }
              }
            }
          }
          frame " INSTRUMENT " {
            n1810 = case shown="\"Cam 1\"" "TabInstrumento" {
              frame "Casseg." {
                w2324 = u16 13 items=["Alarme", "Atencao", "Erro", "Ocupado", "PosSecund", "PosConj#3", "MovFoco", "MovCjto#3", "Mov#4", "Mov#3", "Mov#2", "EspLamp", "HE", "NE", "EspLampRepouso", "EspLampCalibra"] ("NomeStatus")
                w2323 = u16 12 items=["Alarme", "Atencao", "Erro", "Ocupado", "PosSecund", "PosConj#3", "MovFoco", "MovCjto#3", "Mov#4", "Mov#3", "Mov#2", "EspLamp", "HE", "NE", "EspLampRepouso", "EspLampCalibra"] ("NomeStatus")
                w2325 = u16 15 items=["Alarme", "Atencao", "Erro", "Ocupado", "PosSecund", "PosConj#3", "MovFoco", "MovCjto#3", "Mov#4", "Mov#3", "Mov#2", "EspLamp", "HE", "NE", "EspLampRepouso", "EspLampCalibra"] ("NomeStatus")
                w2326 = u16 14 items=["Alarme", "Atencao", "Erro", "Ocupado", "PosSecund", "PosConj#3", "MovFoco", "MovCjto#3", "Mov#4", "Mov#3", "Mov#2", "EspLamp", "HE", "NE", "EspLampRepouso", "EspLampCalibra"] ("NomeStatus")
                w2327 = u16 11 items=["Alarme", "Atencao", "Erro", "Ocupado", "PosSecund", "PosConj#3", "MovFoco", "MovCjto#3", "Mov#4", "Mov#3", "Mov#2", "EspLamp", "HE", "NE", "EspLampRepouso", "EspLampCalibra"] ("NomeStatus")
                # "Cassegrain"
                n1811 = event shown="[3] \"Sent_EspLampCass\": Value Change" {
                  selector: _ -> [_ _ _ _]
                  dyn-events: _ -> [_ _ _ _]
                  timeout: 10 -> [_ _ _ _]
                  event Timeout {
                    n1812 = event-data() -> ()  [unwired: 1 in, 2 out]
                  }
                  event "Ne": Value Change {
                    w2354 = u16 3 items=["ZERO", "AH", "DEC", "TUBO", "CUP"] ("Controlador")
                    n1813 = event-data() -> ()  [unwired: 1 in, 1 out]
                    n1814 = case shown="True" "Ne" {
                      tunnel: ["LAMP_NE" "LAMP_NE"] -> w2353
                      tunnel: ["DESLIGAR" "LIGAR"] -> w2352
                      frame False {
                      }
                      frame True {
                      }
                    }
                    n1815 = call "Monta Comando.vi"("Comando"=w2352, "Dispositivo"=w2353, "Controlador"=w2354) -> ()  [unwired: 4 in, 3 out]
                  }
                  event "He-Ar": Value Change {
                    w2362 = u16 3 items=["ZERO", "AH", "DEC", "TUBO", "CUP"] ("Controlador")
                    n1816 = event-data() -> ()  [unwired: 1 in, 1 out]
                    n1817 = case shown="False" "He-Ar" {
                      tunnel: ["LAMP_HE" "LAMP_HE"] -> w2361
                      tunnel: ["DESLIGAR" "LIGAR"] -> w2360
                      frame False {
                      }
                      frame True {
                      }
                    }
                    n1818 = call "Monta Comando.vi"("Comando"=w2360, "Dispositivo"=w2361, "Controlador"=w2362) -> ()  [unwired: 4 in, 3 out]
                  }
                  event "Sent_EspLampCass": Value Change {
                    w2370 = u16 3 items=["ZERO", "AH", "DEC", "TUBO", "CUP"] ("Controlador")
                    n1819 = event-data() -> ()  [unwired: 1 in, 1 out]
                    n1820 = property on="SlideEcass" class="Slide (strict)"("Visible"=TRUE) -> ()  [unwired: 2 in, 2 out]
                    n1821 = case shown="False" "Sent_EspLampCass" {
                      tunnel: ["ESP_LAMP" "ESP_LAMP"] -> w2369
                      tunnel: ["RECUAR" "AVANCAR"] -> w2368
                      frame False {
                      }
                      frame True {
                      }
                    }
                    n1822 = property on="stopEcass" class="Bool"("Visible"=FALSE) -> ()  [unwired: 2 in, 2 out]
                    n1823 = call "Monta Comando.vi"("Comando"=w2368, "Dispositivo"=w2369, "Controlador"=w2370) -> ()  [unwired: 4 in, 3 out]
                    "SlideEcass" <- u8 8 ("Slide")
                  }
                }
                n1824 = call "Bit Status TUBO.vi"("NomeStatus"=w2323) -> ("StatBit"=→"LedHe":bool)
                n1825 = call "Bit Status TUBO.vi"("NomeStatus"=w2324) -> ("StatBit"=→"LedNe":bool)
                n1826 = call "Bit Status TUBO.vi"("NomeStatus"=w2327) -> ("StatBit"=w2322:bool)
                n1827 = call "Bit Status TUBO.vi"("NomeStatus"=w2326) -> ("StatBit"=w2321:bool)
                n1828 = call "Bit Status TUBO.vi"("NomeStatus"=w2325) -> ("StatBit"=w2320:bool)
                n1829 = And(x=w2322, y=w2321) -> (x .and. y?=w2319:bool)
                "LedRep" <- w2319
                n1830 = And(x=w2322, y=w2320) -> (x .and. y?=w2318:bool)
                "LedCal" <- w2318
                n1831 = property on="SlideEcass" class="Slide (strict)"() -> ("Visible"=w2317:bool)  [unwired: 2 in, 2 out]
                n1832 = Or(x=w2319, y=w2318) -> (x .or. y?=w2329:bool)
                n1833 = Or(x=w2321, y=w2320) -> (x .or. y?=w2332:bool)
                n1834 = Not(x=w2322) -> (.not. x?=w2331:bool)
                n1835 = And(x=w2317, y=w2329) -> (x .and. y?=w2328:bool)
                n1836 = And(x=w2331, y=w2332) -> (x .and. y?=w2330:bool)
                n1837 = case shown="True" w2328 {
                  frame False {
                  }
                  frame True {
                    w2350 = u8 0 ("Disabled")
                    n1838 = property on="Sent_EspLampCass" class="Bool (strict)"("Disabled"=w2350) -> ()  [unwired: 2 in, 2 out]
                    n1839 = property on="He-Ar" class="Bool (strict)"("Disabled"=w2350) -> ()  [unwired: 2 in, 2 out]
                    n1840 = property on="Ne" class="Bool (strict)"("Disabled"=w2350) -> ()  [unwired: 2 in, 2 out]
                    n1841 = property on="SlideEcass" class="Slide (strict)"("Visible"=FALSE) -> ()  [unwired: 2 in, 2 out]
                  }
                }
                n1842 = case shown="True" w2330 {
                  frame False {
                  }
                  frame True {
                    w2334 = u8 2 ("Disabled")
                    n1843 = local read "SlideEcass"() -> (w2335:u8)
                    n1844 = property on="Sent_EspLampCass" class="Bool (strict)"("Disabled"=w2334) -> ()  [unwired: 2 in, 2 out]
                    n1845 = property on="Ne" class="Bool (strict)"("Disabled"=w2334) -> ()  [unwired: 2 in, 2 out]
                    n1846 = property on="He-Ar" class="Bool (strict)"("Disabled"=w2334) -> ()  [unwired: 2 in, 2 out]
                    n1847 = Add(x=w2335, y=u8 4) -> (x+y=w2337:u8)
                    n1848 = Greater Or Equal?(x=w2337, y=u8 100 ("x")) -> (x >= y?=w2338:bool)
                    n1849 = case shown="True" w2338 {
                      selector: w2338 -> [_ w2342]
                      tunnel: w2337 -> [w2341 _]
                      frame False {
                        n1850 = local write "SlideEcass"(w2341) -> ()
                        n1851 = property on="SlideEcass" class="Slide (strict)"("Fill Color"=u32 16750950 ("color(black)")) -> ()  [unwired: 2 in, 2 out]
                      }
                      frame True {
                        n1852 = local write "SlideEcass"(u8 92 ("Slide")) -> ()
                        n1853 = property on="stopEcass" class="Bool"("Visible"=w2342) -> ()  [unwired: 2 in, 2 out]
                        n1854 = property on="SlideEcass" class="Slide (strict)"("Fill Color"=u32 16724787 ("color(black)")) -> ()  [unwired: 2 in, 2 out]
                      }
                    }
                  }
                }
                n1855 = case shown="True" "stopEcass" {
                  frame False {
                  }
                  frame True {
                    w2349 = FALSE
                    w2348 = u8 0 ("Disabled")
                    w2347 = u16 3 items=["ZERO", "AH", "DEC", "TUBO", "CUP"] ("Controlador")
                    n1856 = call "Monta Comando.vi"("Comando"="DESLIGAR", "Dispositivo"="ESP_LAMP", "Controlador"=w2347) -> ()  [unwired: 4 in, 3 out]
                    n1857 = property on="Sent_EspLampCass" class="Bool (strict)"("Disabled"=w2348) -> ()  [unwired: 2 in, 2 out]
                    n1858 = property on="Ne" class="Bool (strict)"("Disabled"=w2348) -> ()  [unwired: 2 in, 2 out]
                    n1859 = property on="He-Ar" class="Bool (strict)"("Disabled"=w2348) -> ()  [unwired: 2 in, 2 out]
                    n1860 = property on="SlideEcass" class="Slide (strict)"("Visible"=w2349) -> ()  [unwired: 2 in, 2 out]
                    n1861 = property on="stopEcass" class="Bool"("Visible"=w2349) -> ()  [unwired: 2 in, 2 out]
                  }
                }
              }
              frame "Eucalyp." {
                # "Eucalyptus"
              }
              frame "Cam 1" {
                w2386 = 10
                w2393 = u16 15 items=["Alarme", "Atencao", "Erro", "Ocupado", "PosSecund", "PosConj#3", "MovFoco", "MovCjto#3", "Mov#4", "Mov#3", "Mov#2", "EspLamp", "HE", "NE", "EspLampRepouso", "EspLampCalibra"] ("NomeStatus")
                w2394 = u16 14 items=["Alarme", "Atencao", "Erro", "Ocupado", "PosSecund", "PosConj#3", "MovFoco", "MovCjto#3", "Mov#4", "Mov#3", "Mov#2", "EspLamp", "HE", "NE", "EspLampRepouso", "EspLampCalibra"] ("NomeStatus")
                w2395 = u16 11 items=["Alarme", "Atencao", "Erro", "Ocupado", "PosSecund", "PosConj#3", "MovFoco", "MovCjto#3", "Mov#4", "Mov#3", "Mov#2", "EspLamp", "HE", "NE", "EspLampRepouso", "EspLampCalibra"] ("NomeStatus")
                # "MUDANÇA:\nDESABILITA COMANDOS\nDE MOV. DO ESPELHO.\nRemover na implantação\ndefinitiva da CAM1."
                # "CAM 1"
                n1862 = event shown="[0] Timeout" {
                  selector: _ -> [_ _ _ _]
                  dyn-events: _ -> [_ _ _ _]
                  timeout: w2386 -> [_ _ _ _]
                  tunnel: ["timeout" ("Comando") w2412 w2418 w2424] -> w2379
                  event Timeout {
                    n1863 = event-data() -> ()  [unwired: 1 in, 2 out]
                  }
                  event "Mover/Parar": Value Change {
                    w2414 = u16 3 items=["ZERO", "AH", "DEC", "TUBO", "CUP"] ("Controlador")
                    n1864 = event-data() -> ("NewVal"=w2415:bool)  [unwired: 1 in, 4 out]
                    n1865 = case shown="True" w2415 {
                      tunnel: ["PARAR" ("Comando") "GIRAR" ("Comando")] -> w2412
                      frame False {
                      }
                      frame True {
                      }
                    }
                    n1866 = call "Monta Comando.vi"("Comando"=w2412, "Dispositivo"="ESP_CAMP", "Controlador"=w2414) -> ()  [unwired: 4 in, 3 out]
                  }
                  event "Sentido": Value Change {
                    w2419 = u16 3 items=["ZERO", "AH", "DEC", "TUBO", "CUP"] ("Controlador")
                    n1867 = event-data() -> ("NewVal"=w2421:bool)  [unwired: 1 in, 4 out]
                    n1868 = case shown="False" w2421 {
                      tunnel: ["RECUAR" "AVANCAR"] -> w2418
                      frame False {
                      }
                      frame True {
                      }
                    }
                    n1869 = call "Monta Comando.vi"("Comando"=w2418, "Dispositivo"="ESP_CAMP", "Controlador"=w2419) -> ()  [unwired: 4 in, 3 out]
                  }
                  event "Velocidade": Value Change {
                    w2426 = u16 3 items=["ZERO", "AH", "DEC", "TUBO", "CUP"] ("Controlador")
                    n1870 = event-data() -> ("NewVal"=w2427:bool)  [unwired: 1 in, 4 out]
                    n1871 = case shown="True" w2427 {
                      tunnel: ["AUMENTAR" "DIMINUIR"] -> w2424
                      frame False {
                      }
                      frame True {
                      }
                    }
                    n1872 = call "Monta Comando.vi"("Comando"=w2424, "Dispositivo"="ESP_CAMP", "Controlador"=w2426) -> ()  [unwired: 4 in, 3 out]
                  }
                }
                "Comando" <- w2379
                n1873 = case shown="False" "Sentido" {
                  tunnel: [TRUE FALSE] -> w2384
                  tunnel: [FALSE TRUE] -> w2383
                  frame False {
                  }
                  frame True {
                  }
                }
                "Recuar" <- w2384
                "Avancar" <- w2383
                n1874 = event shown="[1] \"Sent_EspDesvFeixe\": Value Change" {
                  selector: _ -> [_ _ _]
                  dyn-events: _ -> [_ _ _]
                  timeout: w2386 -> [_ _ _]
                  event Timeout {
                    n1875 = event-data() -> ()  [unwired: 1 in, 2 out]
                  }
                  event "Sent_EspDesvFeixe": Value Change {
                    n1876 = event-data() -> ()  [unwired: 1 in, 4 out]
                    n1877 = case shown="1" "Disabled" {
                      tunnel: ["RECUAR" ("Comando") "AVANCAR" ("Comando")] -> w2433
                      tunnel: ["ESP_LAMP" ("Dispositivo") "ESP_LAMP" ("Dispositivo")] -> w2432
                      frame 0, Default {
                        # "Case False (Default) em\noperação normal, com o\nbotão Sent_EspDesvFeixe\nligado ao ? deste case."
                      }
                      frame 1 {
                        # "CaseTrue. Cf. nota no case 0"
                        n1878 = property on="SlideCam1" class="Slide (strict)"("Visible"=TRUE) -> ()  [unwired: 2 in, 2 out]
                        n1879 = property on="stopCam1" class="Bool"("Visible"=FALSE) -> ()  [unwired: 2 in, 2 out]
                        "SlideCam1" <- u8 5 ("Slide 2")
                      }
                    }
                    n1880 = case shown="True" "Case Constant\n(See Context Help) 9" {
                      tunnel: w2433 -> [_ w2436]
                      tunnel: w2432 -> [_ w2435]
                      frame False {
                      }
                      frame True {
                        w2434 = u16 3 items=["ZERO", "AH", "DEC", "TUBO", "CUP"] ("Controlador")
                        n1881 = call "Monta Comando.vi"("Comando"=w2436, "Dispositivo"=w2435, "Controlador"=w2434) -> ()  [unwired: 4 in, 3 out]
                      }
                    }
                  }
                  event "Go_filtro": Value Change {
